vi "IPS Current Sweep Rate Amp per min.vi"(3 "Error In":errorcluster={"status"=FALSE, "code"=1073676294, "source"="VISA Read in Prologix USB GPIB Command.vi"}, 4 "Field Sweep Rate (T/min)":dbl min=-0.2 max=0.2, 5 "VISA resource name (COM Port of Prologix Device)":refnum<visa-resource-name>="COM3") -> (0 "Error Out":errorcluster={"status"=FALSE, "code"=1073676294, "source"="VISA Read in Prologix_GPIB_Sample.vi"}, 2 "Output":string)   [LabVIEW 2011]
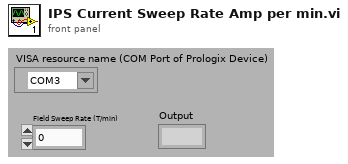
[diagram p1: front panel]
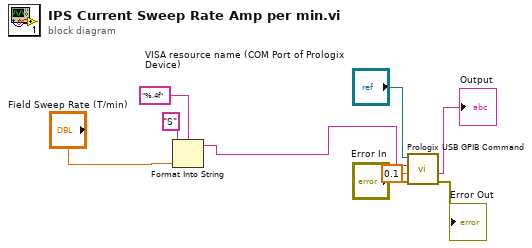
[diagram p0: block diagram]
diagram:
  n1 = Format Into String(format string="%.4f", initial string="S" ("string (\"\")"), "Field Sweep Rate (T/min)") -> (resulting string=w1:string)  [unwired: 1 in, 1 out]
  n2 = call <userlib>:"Prologix USB GPIB Command.vi"("Error In"="Error In", "Wait for instrument to respond (s)"=0.1, "String to Send"=w1, "VISA resource name (COM Port of Prologix Device)"="VISA resource name (COM Port of Prologix Device)") -> ("Error Out"=→"Error Out":errorcluster, "Return String from Device (Not all commands return a String)"=→"Output":string)  [unwired: 2 out]
